vi "Toggle.vi"(8 "Error In":errorcluster, 11 "Button Input":bool) -> (0 "Error Out":errorcluster, 3 "Toggle Output":bool)   [LabVIEW 2014]
doc: "When Button Input registers \"True\", Toggle Output switches state. This function prevents repeated \"True\" inputs from switching the state more than once. This may occur if the driver or operator holds down a button, thoug only intends to change state once."
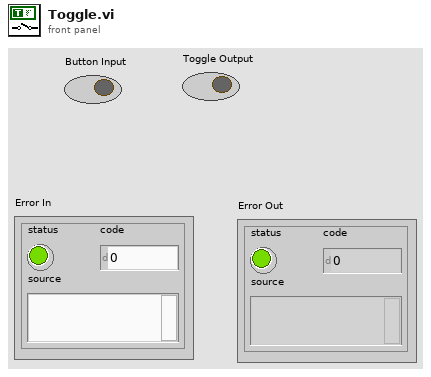
[diagram p1: front panel]
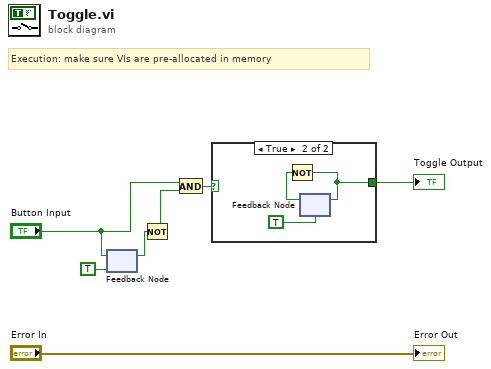
[diagram p0: block diagram]
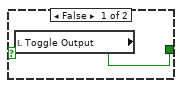
[diagram p2: hidden frame]
diagram:
  # "Execution: make sure VIs are pre-allocated in memory"
  n1 = feedback #1(TRUE) -> (w4:bool)
  n2 = feedback-in #1("Button Input") -> ()
  n3 = Not(x=w4) -> (.not. x?=w5:bool)
  n4 = And(x="Button Input", y=w5) -> (x .and. y?=w6:bool)
  n5 = case shown="True" w6 {
    tunnel: [w8 w9] -> w7
    frame False {
      n6 = local read "Toggle Output"() -> (w8:bool)
    }
    frame True {
      n7 = feedback #2(TRUE) -> (w10:bool)
      n8 = Not(x=w10) -> (.not. x?=w9:bool)
      n9 = feedback-in #2(w9) -> ()
    }
  }
  "Toggle Output" <- w7
  "Error Out" <- "Error In"
